vi "Divide Vector by Scalar - Return 1D Array.vi"(1 "Vector":T1 format="%_8f", 4 "x":dbl format="%_8f") -> (15 "Scaled (1D)-Array":dbl[](array[numeric]) format="%_8g")   [LabVIEW 2014]
uses:
  <vilib>/Analysis/Matrix/Datatypes/RealMatrix.ctl
  <vilib>/Analysis/Matrix/NI_Matrix.lvlib
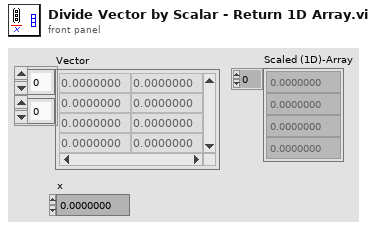
[diagram p1: front panel]
types:
  T1 = typedef "NI_Matrix.lvlib/RealMatrix.ctl" = dbl[][]
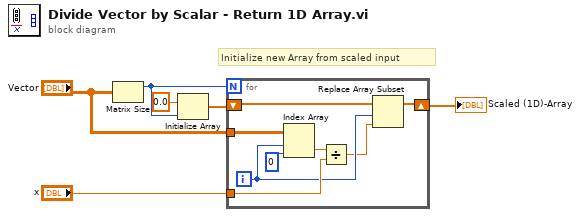
[diagram p0: block diagram]
diagram:
  # "Initialize new Array from scaled input"
  n1 = Matrix Size(0:"Vector") -> (1:w4:i32)  [unwired: 1 out]
  n2 = Initialize Array(0.0 ("element"), w4) -> (w2:dbl[])
  n3 = for {
    N: w4 -> [_]
    tunnel: "Vector" -> [w14]
    shift-right: [w7] -> w1
    shift-left: w2 -> [w10]
    tunnel: "x" -> [w11]
    i -> [w9]
    n4 = Index Array(array=w14, index (row)=w9, index (col)=0) -> (element=w12:dbl)
    n5 = Divide(x=w12, y=w11) -> (x/y=w8:dbl)
    n6 = Replace Array Subset(array=w10, new element=w8, index=w9) -> (w7:dbl[])
  }
  "Scaled (1D)-Array" <- w1
